vi "Apply Branding.vi"(8 "error in (no error)":errorcluster, 11 "Main in":refnum<class "Main.lvclass">) -> (0 "error out":errorcluster, 3 "Main out":refnum<class "Main.lvclass">)   [LabVIEW 2023, in "Main.lvlib" / "Main.lvclass"]
uses:
  Library/Main.lvclass
  C:/Users/Public/Documents/Development/builds/Framework/Engine.lvlibp/Engine/Library/Engine.lvclass
  Library/Main.lvclass/Main.ctl
  builds/Framework/Engine.lvlibp/Engine/Accessors/Read Application Path.vi
  builds/Tools/EmbedImage.lvlibp/Library/EmbedImage.lvclass
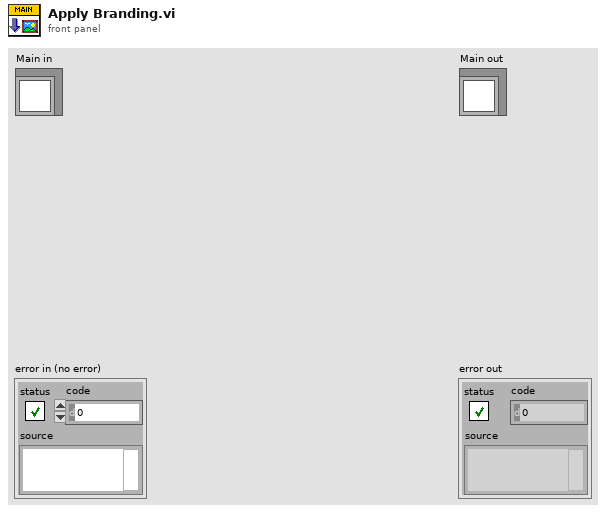
[diagram p1: front panel]
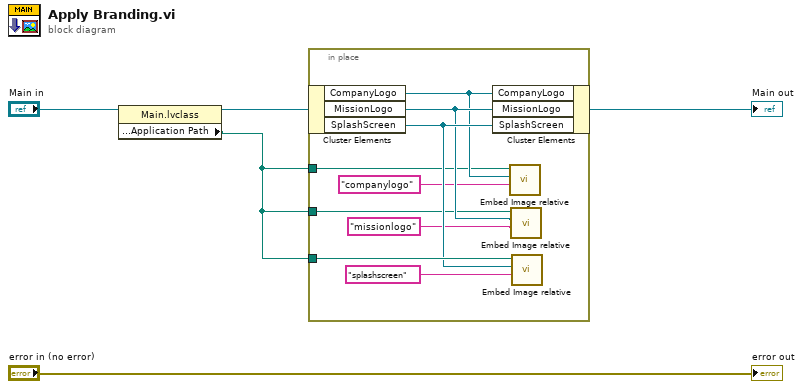
[diagram p0: block diagram]
diagram:
  n1 = property class="Main.lvclass"(reference="Main in") -> (reference out=w2:refnum<class "Main.lvclass">, "Accessors:Configuration:Application Path"=w1:path)  [unwired: 1 in, 1 out]
  n2 = in-place {
    in-place-border: w1 -> [w6]
    in-place-border: w1 -> [w9]
    in-place-border: w1 -> [w14]
    n3 = in-place-cluster #1(w2) -> ("CompanyLogo"=w7:refnum<vi>, "MissionLogo"=w10:refnum<vi>, "SplashScreen"=w13:refnum<vi>)
    n4 = in-place-cluster #1("CompanyLogo"=w7, "MissionLogo"=w10, "SplashScreen"=w13) -> (→"Main out":refnum<class "Main.lvclass">)
    n5 = call "Embed Image relative.vi"("imagename"="companylogo" ("ImageName"), "Pict Refnum"=w7, "Application path"=w6) -> ()  [unwired: 8 in, 1 out]
    n6 = call "Embed Image relative.vi"("imagename"="missionlogo" ("ImageName"), "Pict Refnum"=w10, "Application path"=w9) -> ()  [unwired: 8 in, 1 out]
    n7 = call "Embed Image relative.vi"("imagename"="splashscreen" ("ImageName"), "Pict Refnum"=w13, "Application path"=w14) -> ()  [unwired: 8 in, 1 out]
  }
  "error out" <- "error in (no error)"
